vi "PathPlanner_PointTowardsZone_Equals.vi"(9 "OtherPointTowardsZone":T1={"RotationOffset"={"VALUE"=0.0, "COS"=1.0, "SIN"=0.0}, "Name"="", "TargetPosition"={"X"=0.0, "Y"=0.0}, "MinPosition"=0.0, "MaxPosition"=0.0} {"TargetPosition"."Y" format="%14.3f"; "TargetPosition"."X" format="%14.3f"; "RotationOffset"."SIN" format="%13.4f"; "RotationOffset"."COS" format="%13.4f"; "RotationOffset"."VALUE" format="%13.4f"}, 11 "PointTowardsZone":T1={"RotationOffset"={"VALUE"=0.0, "COS"=1.0, "SIN"=0.0}, "Name"="", "TargetPosition"={"X"=0.0, "Y"=0.0}, "MinPosition"=0.0, "MaxPosition"=0.0} {"TargetPosition"."Y" format="%14.3f"; "TargetPosition"."X" format="%14.3f"; "RotationOffset"."SIN" format="%13.4f"; "RotationOffset"."COS" format="%13.4f"; "RotationOffset"."VALUE" format="%13.4f"}) -> (3 "Equals":bool)   [LabVIEW 2019, in "PathPlanner24.lvlib"]
doc: "Create a new rotation target\n\nInputs: \n - position - double - Waypoint relative position of this target\n - rotation - rotation2d - Target rotation\n\nOutputs:\n - RotationTarget - cluster - defined rotation target data structure"
uses:
  TypeDef/PathPlannerPointTowardsZone.ctl
  <vilib>/Rock Robotics/WPI/ThirdParty/JAS_Junk/TrajLib/TypeDef/ROTATION2D.ctl
  <vilib>/Rock Robotics/WPI/ThirdParty/JAS_Junk/TrajLib/TypeDef/TRANSLATION2D.ctl
  PathPlanner_FieldUtil_SymmetryType.vi
  PathPlanner_FieldUtil_FieldSizeY.vi
  <vilib>/Rock Robotics/WPI/ThirdParty/JAS_Junk/TrajLib/Translation2d_GetXY.vi
  <vilib>/Rock Robotics/WPI/ThirdParty/JAS_Junk/TrajLib/Translation2d_Create.vi
  PathPlanner_FieldUtil_FieldSizeX.vi
  <vilib>/Rock Robotics/WPI/ThirdParty/JAS_Junk/TrajLib/Conv_Feet_Meters.vi
  PathPlanner24.lvlib
  <vilib>/Rock Robotics/WPI/ThirdParty/JAS_Junk/TrajLib/Trajectory_Library.lvlib
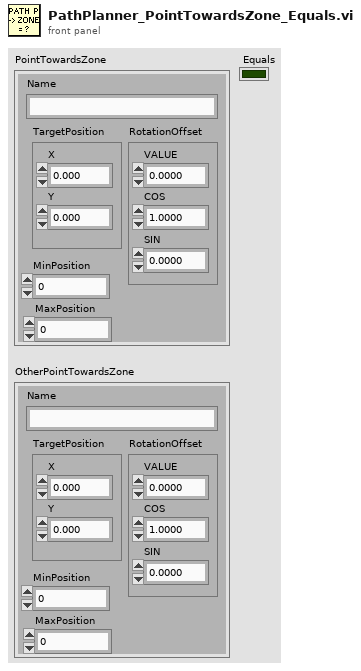
[diagram p1: front panel]
types:
  T1 = typedef "PathPlanner24.lvlib/PathPlannerPointTowardsZone.ctl" = cluster{"RotationOffset":T2, "Name":string, "TargetPosition":T3, "MinPosition":dbl, "MaxPosition":dbl}
  T2 = typedef "Trajectory_Library.lvlib/ROTATION2D.ctl" = cluster{"VALUE":dbl, "COS":dbl, "SIN":dbl}
  T3 = typedef "Trajectory_Library.lvlib/TRANSLATION2D.ctl" = cluster{"X":dbl, "Y":dbl}
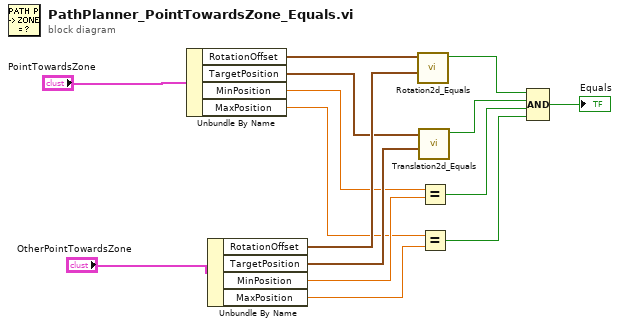
[diagram p0: block diagram]
diagram:
  n1 = Unbundle By Name("PointTowardsZone") -> ("RotationOffset"=w13:T2, "TargetPosition"=w11:T3, "MinPosition"=w5:dbl, "MaxPosition"=w3:dbl)
  n2 = Unbundle By Name("OtherPointTowardsZone") -> ("RotationOffset"=w12:T2, "TargetPosition"=w10:T3, "MinPosition"=w4:dbl, "MaxPosition"=w2:dbl)
  n3 = call <vilib>:"Rotation2d_Equals.vi"("other ROTATION"=w12, "in ROTATION"=w13) -> ("Equals"=w9:bool)  [unwired: 9 in]
  n4 = call <vilib>:"Translation2d_Equals.vi"("other Translation"=w10, "In Translation"=w11) -> ("Equals"=w8:bool)  [unwired: 9 in]
  n5 = Equal?(x=w5, y=w4) -> (x = y?=w7:bool)
  n6 = Equal?(x=w3, y=w2) -> (x = y?=w6:bool)
  n7 = Compound Arithmetic op=AND(w9, w8, w7, w6) -> (→"Equals":bool)
